vi "zmq_unbind.vi"(3 "error in":errorcluster, 4 "endpoint":string, 5 "socket in":refnum<class "zmq_socket.lvclass">) -> (0 "error out":errorcluster, 2 "socket out":refnum<class "zmq_socket.lvclass">)   [LabVIEW 2020, in "zeromq.lvlib" / "zmq_socket.lvclass"]
doc: "Unbinds a socket from a particular <b>endpoint</b>. Opposite of zmq_bind. Use zmq_close to unbind from all endpoints.\n\nDetailed API documentation: http://api.zeromq.org/3-2:zmq-unbind"
uses:
  zmq_socket.lvclass
  zmq_socket.lvclass/zmq_socket.ctl
  Error Cluster From Error Code.vi
  zeromq.lvlib
panel:
  # "ØMQ"
  # "labview"
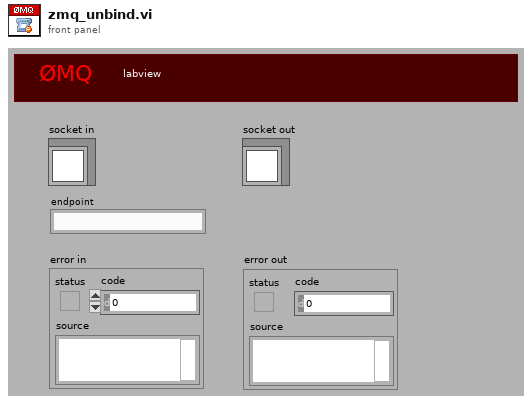
[diagram p1: front panel]
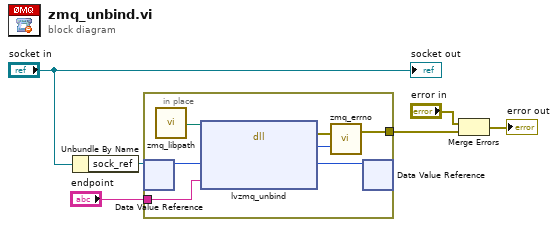
[diagram p0: block diagram]
diagram:
  n1 = Unbundle By Name("socket in") -> ("sock_ref"=w3:refnum<data-value>)
  n2 = in-place {
    in-place-border: "endpoint" -> [w13]
    in-place-border: [w10] -> w5
    n3 = in-place-dvr #1(w3) -> (w9:u64)  [unwired: 1 out]
    n4 = call "zmq_libpath.vi"() -> ("path"=w7:path)
    n5 = dll-call lib="?" fn="lvzmq_unbind" ("zmq_labview.dll:lvzmq_bind")(path in=w7, "sock_obj"=w9, "endpoint"=w13) -> (error out=w12:errorcluster, "return type"=w11:i32, "sock_obj"=w8:u64)  [unwired: 3 in, 1 out]
    n6 = call "zmq_errno.vi"("retval"=w11, "error in"=w12) -> ("error out"=w10:errorcluster)  [unwired: 1 out]
    n7 = in-place-dvr #1(w8) -> ()  [unwired: 2 out]
  }
  n8 = Merge Errors("error in", w5) -> (→"error out":errorcluster)
  "socket out" <- "socket in"
